vi "Set Payload.vi"(8 "error in (no error)":errorcluster, 10 "Payload":string, 11 "Response in":refnum<class "Response.lvclass">) -> (0 "error out":errorcluster, 3 "Response out":refnum<class "Response.lvclass">)   [LabVIEW 2020, in "HTTP Utils.lvlib" / "Response.lvclass"]
uses:
  Response.lvclass
  Response.lvclass/Response.ctl
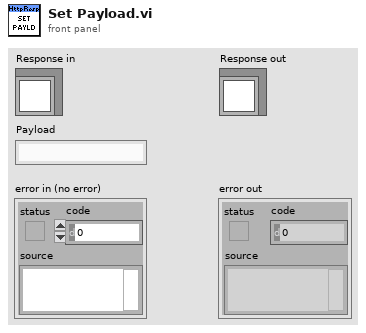
[diagram p1: front panel]
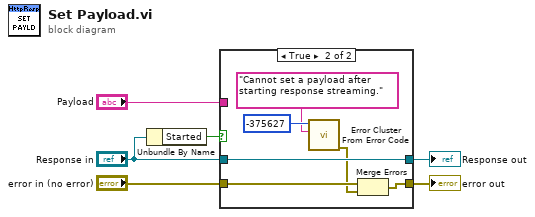
[diagram p0: block diagram]
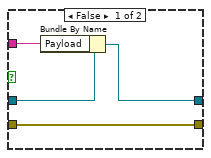
[diagram p2: hidden frame]
diagram:
  n1 = Unbundle By Name("Response in") -> ("Started"=w3:bool)
  n2 = case shown="True" w3 {
    tunnel: [w10 w16] -> w6
    tunnel: "Payload" -> [w9 _]
    tunnel: "Response in" -> [w8 w16]
    tunnel: "error in (no error)" -> [w7 w15]
    tunnel: [w7 w14] -> w1
    frame False {
      n3 = Bundle By Name(cluster=w8, "Payload"=w9) -> (w10:refnum<class "Response.lvclass">)
    }
    frame True {
      n4 = call <vilib>:"Error Cluster From Error Code.vi"("error message (\"\")"="Cannot set a payload after starting response streaming." ("error message (\"\")"), "error code (0)"=-375627) -> ("error out"=w11:errorcluster)  [unwired: 7 in]
      n5 = Merge Errors(w15, w11) -> (w14:errorcluster)
    }
  }
  "error out" <- w1
  "Response out" <- w6
